vi "Funktionsgenerator ohne Demod.vi"() -> ()   [LabVIEW 2017]
uses:
  <vilib>/Utility/error.llb/DialogType.ctl
  <vilib>/DAQmx/read.llb/DAQmx Read (Analog Wfm 1Chan NSamp).vi
  <vilib>/DAQmx/create/channels.llb/DAQmx Create Channel (AI-Voltage-Basic).vi
  <vilib>/DAQmx/configure/timing.llb/DAQmx Timing (Sample Clock).vi
  <vilib>/DAQmx/miscellaneous.llb/DAQmx Fill In Error Info.vi
  <vilib>/express/express analysis/Spectral/Block/exnSpectralBlock spectral measurements power poly.vi
  <vilib>/express/express analysis/Spectral/Block/exnSpectralBlock spectral measurements power WFM.vi
  <vilib>/Utility/file.llb/Write Delimited Spreadsheet (DBL).vi
  <vilib>/express/express analysis/Spectral/XNode/ExpressSpectralMeasurementsBlockNode.xnode
panel:
  in  "Speichern":bool
  out "Spektrum mit Hann-Fenster":cluster{"f0":dbl, "df":dbl, "magnitude":dbl[]}(graph)
  out "Spektrum ohne Hann-Fenster":cluster{"f0":dbl, "df":dbl, "magnitude":dbl[]}(graph)
  in  "stop":bool
  out "Zeitlicher Verlauf":waveform(dbl)(graph)
  in  "minimum value":dbl=-5.0 format="%0.2f"
  in  "maximum value":dbl=5.0 format="%0.2f"
  in  "rate":dbl=1000.0 format="%0.2f"
  in  "physical channels":tag
  in  "samples per channel":i32=1000
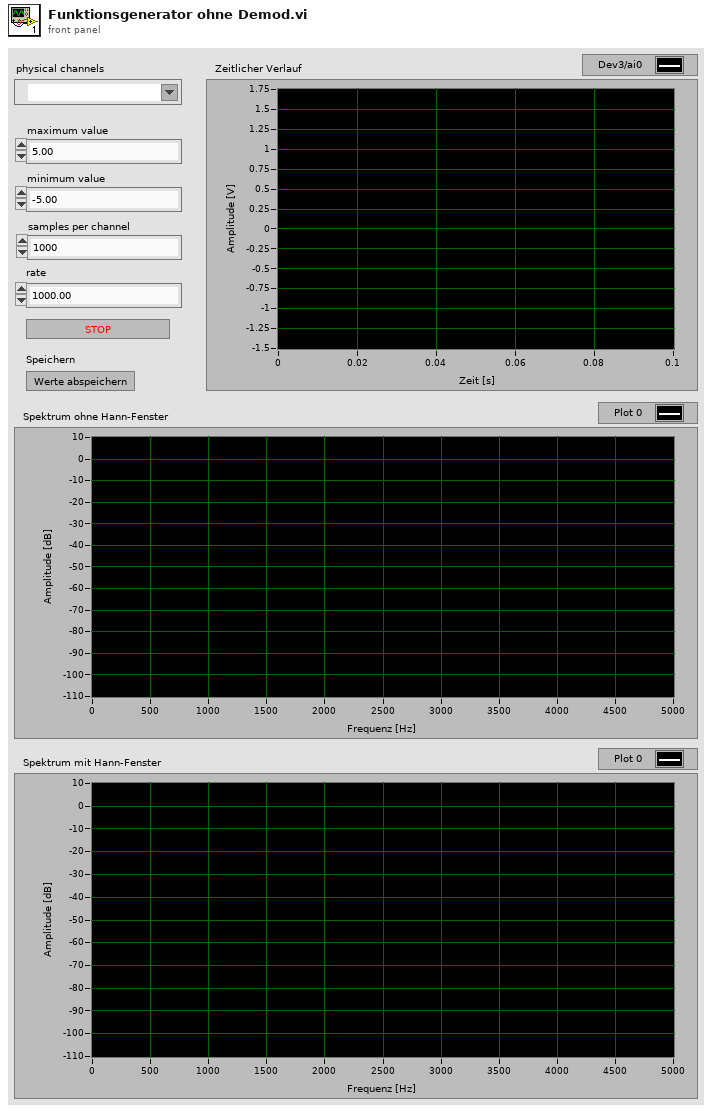
[diagram p1: front panel]
types:
  T1 = cluster{"averaging mode":u16, "weighting mode":u16, "number of averages":u32}
  T2 = cluster{"dB On (F)":bool, "unwrap phase (F)":bool, "convert to degree (F)":bool}
  T3 = typedef "DialogType.ctl" = u16
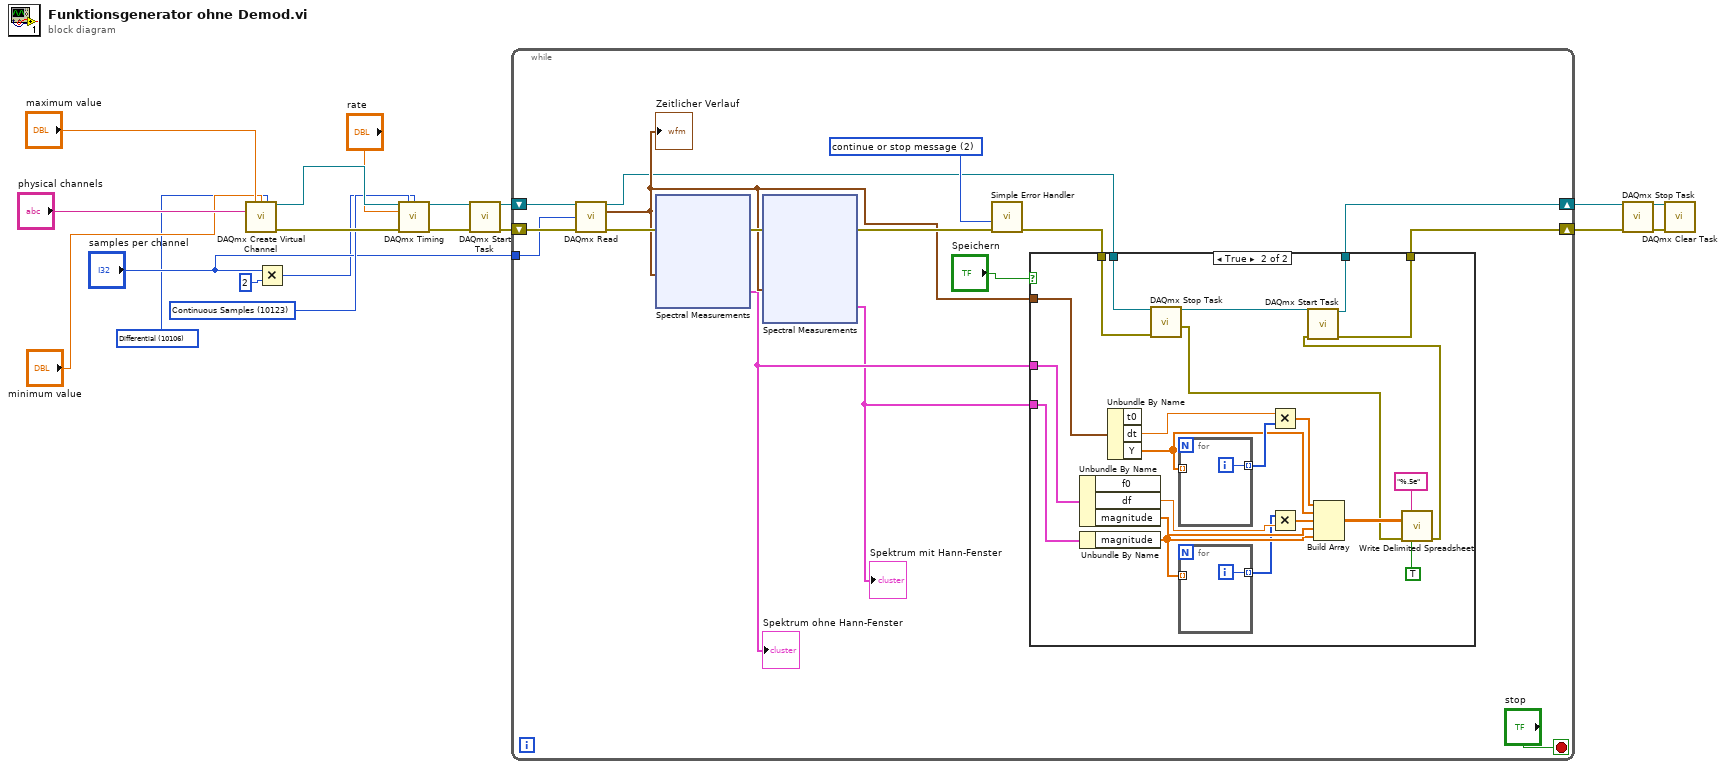
[diagram p0: block diagram]
diagram:
  w5 = 10123 items=["Finite Samples"=10178, "Continuous Samples"=10123, "Hardware Timed Single Point"=12522] ("sample mode")
  w3 = 10106 items=["Default"=-1, "RSE"=10083, "NRSE"=10078, "Differential"=10106, "Pseudodifferential"=12529] ("input terminal configuration")
  n1 = call-poly <vilib>:"DAQmx Create Virtual Channel.vi"("maximum value"="maximum value", "minimum value"="minimum value", "input terminal configuration"=w3, "physical channels"="physical channels") -> ("task out"=w14:refnum<k21>, "error out"=w19:errorcluster)  [unwired: 10 in]
  n2 = Multiply(x="samples per channel", y=2 ("x*y")) -> (x*y=w2:i32)
  n3 = call-poly <vilib>:"DAQmx Timing.vi"("task/channels in"=w14, "sample mode"=w5, "samples per channel"=w2, "rate"="rate", "error in"=w19) -> ("task out"=w13:refnum<k21>, "error out"=w18:errorcluster)  [unwired: 9 in]
  n4 = call <vilib>:"DAQmx Start Task.vi"("task/channels in"=w13, "error in"=w18) -> ("task out"=w12:refnum<k21>, "error out"=w17:errorcluster)  [unwired: 12 in]
  n5 = while {
    shift-right: [w21] -> w16
    shift-left: w17 -> [w35]
    shift-right: [w23] -> w11
    shift-left: w12 -> [w34]
    tunnel: "samples per channel" -> [w32]
    stop <- "stop" stop-if-true
    w31 = T3 2 items=["no dialog", "OK message", "continue or stop message", "OK message + warnings", "continue/stop + warnings"] ("type of dialog (OK msg:1)")
    n6 = call-poly <vilib>:"DAQmx Read.vi"("task/channels in"=w34, "number of samples per channel"=w32, "error in"=w35) -> ("task out"=w24:refnum<k21>, "data"=w27:waveform(dbl), "error out"=w30:errorcluster)  [unwired: 10 in]
    "Zeitlicher Verlauf" <- w27
    n7 = xnode "Spectral Measurements"("Signals"=w27, "error in (no error)"=w30) -> ("Power Spectrum"=w26:cluster{"f0":dbl, "df":dbl, "magnitude":dbl[]}, "error out"=w29:errorcluster)
    "Spektrum ohne Hann-Fenster" <- w26
    n8 = xnode "Spectral Measurements"("Signals"=w27, "error in (no error)"=w29) -> ("Power Spectrum"=w25:cluster{"f0":dbl, "df":dbl, "magnitude":dbl[]}, "error out"=w28:errorcluster)
    "Spektrum mit Hann-Fenster" <- w25
    n9 = call <vilib>:"Simple Error Handler.vi"("type of dialog (OK msg:1)"=w31, "error in (no error)"=w28) -> ("error out"=w22:errorcluster)  [unwired: 3 in, 4 out]
    n10 = case shown="True" "Speichern" {
      tunnel: w27 -> [_ w57]
      tunnel: w26 -> [_ w56]
      tunnel: w25 -> [_ w55]
      tunnel: w24 -> [w37 w44]
      tunnel: [w37 w42] -> w23
      tunnel: w22 -> [w36 w41]
      tunnel: [w36 w38] -> w21
      frame False {
      }
      frame True {
        n11 = Unbundle By Name(w56) -> ("df"=w50:dbl, "magnitude"=w54:dbl[])  [unwired: 1 out]
        n12 = Unbundle By Name(w55) -> ("magnitude"=w48:dbl[])
        n13 = Unbundle By Name(w57) -> ("dt"=w52:dbl, "Y"=w45:dbl[])  [unwired: 1 out]
        n14 = call <vilib>:"DAQmx Stop Task.vi"("task/channels in"=w44, "error in"=w41) -> ("task out"=w43:refnum<k21>, "error out"=w40:errorcluster)  [unwired: 12 in]
        n15 = for {
          tunnel: [w61] -> w49 mode=indexing
          tunnel: w45 -> [_] mode=indexing
          i -> [w61]
        }
        n16 = for {
          tunnel: w48 -> [_] mode=indexing
          tunnel: [w60] -> w47 mode=indexing
          i -> [w60]
        }
        n17 = Multiply(x=w52, y=w49) -> (x*y=w51:dbl[])
        n18 = Multiply(x=w47, y=w50) -> (x*y=w46:dbl[])
        n19 = Build Array(w51, w45, w46, w54, w48) -> (w53:dbl[][])
        n20 = call-poly <vilib>:"Write Delimited Spreadsheet.vi"("format (%.3f)"="%.5e", "2D data"=w53, "error in (no error)"=w40, "transpose? (no:F)"=TRUE) -> ("error out"=w39:errorcluster)  [unwired: 10 in, 1 out]
        n21 = call <vilib>:"DAQmx Start Task.vi"("task/channels in"=w43, "error in"=w39) -> ("task out"=w42:refnum<k21>, "error out"=w38:errorcluster)  [unwired: 12 in]
      }
    }
  }
  n22 = call <vilib>:"DAQmx Stop Task.vi"("task/channels in"=w11, "error in"=w16) -> ("task out"=w10:refnum<k21>, "error out"=w15:errorcluster)  [unwired: 12 in]
  n23 = call <vilib>:"DAQmx Clear Task.vi"("task in"=w10, "error in"=w15) -> ()  [unwired: 13 in, 1 out]
